vi "test Add Invalid Alias.vi"(8 "error in (no error)":errorcluster, 11 "TestCase in":refnum<class "Routing and Faulting Aliases Unit Tests.lvclass">) -> (0 "error out":errorcluster, 3 "TestCase out":refnum<class "Routing and Faulting Aliases Unit Tests.lvclass">)   [LabVIEW 2019, in "Routing and Faulting Aliases Unit Tests.lvclass"]
uses:
  Routing and Faulting Aliases Unit Tests.lvclass
  Shared/Alias Mapping.ctl
  Shared/Alias Endpoint.ctl
  System Explorer/Alias.ctl
  System Explorer/Endpoint.ctl
  Routing and Faulting Aliases Unit Tests.lvclass/Routing and Faulting Aliases Unit Tests.ctl
  <vilib>/addons/_JKI Toolkits/VI Tester/TestCase.llb/TestCase.lvclass
  System Explorer/Routing and Faulting System Explorer.lvlib
  Scripting/Routing and Faulting Scripting.lvlib
  Shared/Routing and Faulting Shared.lvlib
  C:/Program Files (x86)/National Instruments/LabVIEW 2019/vi.lib/addons/_JKI Toolkits/VI Tester/TestCase.llb/TestCase.lvclass
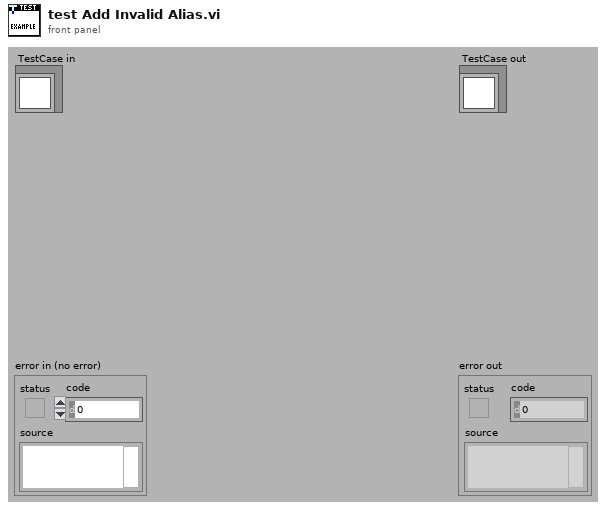
[diagram p1: front panel]
types:
  T1 = typedef "Routing and Faulting Shared.lvlib/Alias Endpoint.ctl" = cluster{"Module Path":string, "Endpoint":string}
  T2 = typedef "Routing and Faulting System Explorer.lvlib/Endpoint.ctl" = string
  T3 = typedef "Routing and Faulting Shared.lvlib/Alias Mapping.ctl" = cluster{"Alias":string, "Endpoint":T1}
  T4 = typedef "Routing and Faulting System Explorer.lvlib/Alias.ctl" = cluster{"Endpoint":T2, "Alias":string, "Remove":bool}
  T5 = typedef "Custom Device API.lvlib/Custom Device Item Ref.ctl" = u64
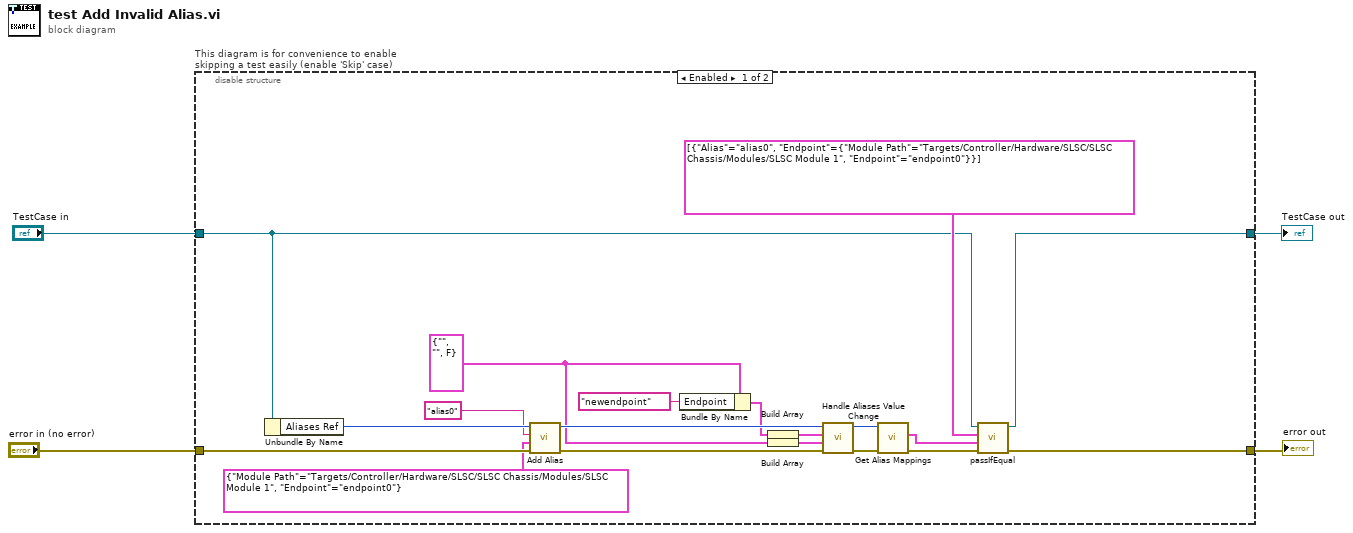
[diagram p0: block diagram]
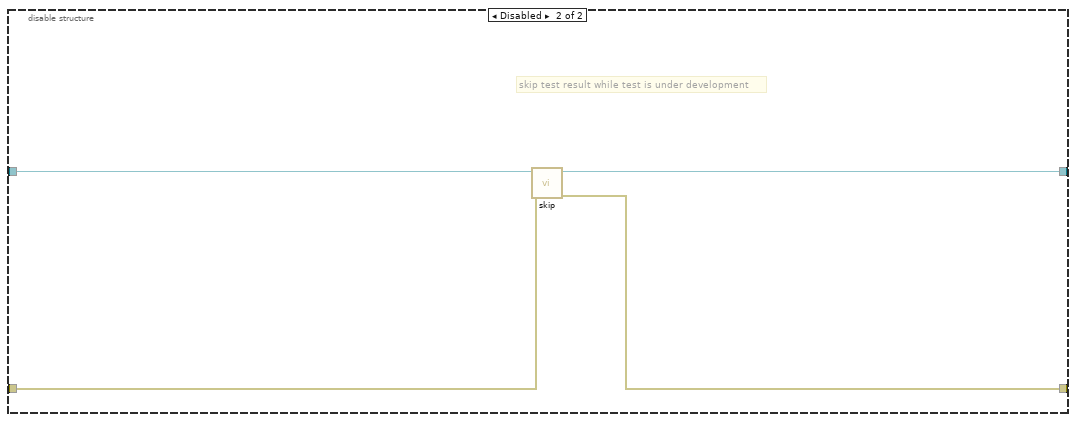
[diagram p2: hidden frame]
diagram:
  n1 = disable-structure "This diagram is for convenience to enable skipping a test easily (enable 'Skip' case)" shown="Enabled" {
    disable-tunnel: "TestCase in" -> [w17 w27]
    disable-tunnel: [w16 w25] -> w1
    disable-tunnel: [w20 w26] -> w3
    disable-tunnel: "error in (no error)" -> [w14 w24]
    frame Enabled {
      w7 = T4 {"Endpoint"="", "Alias"="", "Remove"=FALSE} ("Alias")
      n2 = Unbundle By Name(w17) -> ("Aliases Ref"=w15:T5)
      n3 = call "Add Alias.vi"("error in"=w14, "endpoint"=T1 {"Module Path"="Targets/Controller/Hardware/SLSC/SLSC Chassis/Modules/SLSC Module 1", "Endpoint"="endpoint0"} ("Endpoint"), "alias"="alias0" ("Alias"), "endpoint aliases in"=w15) -> ("error out"=w12:errorcluster, "endpoint aliases out"=w13:T5)  [unwired: 6 in]
      n4 = Bundle By Name(cluster=w7, "Endpoint"=T2 "newendpoint") -> (w8:T4)
      n5 = Build Array(w8) -> (w9:T4[])
      n6 = Build Array(w7) -> (w10:T4[])
      n7 = call "Handle Aliases Value Change.vi"("error in (no error)"=w12, "OldVal"=w10, "NewVal"=w9, "Aliases Ref in"=w13) -> ("error out"=w23:errorcluster, "Aliases Ref out"=w22:T5)  [unwired: 4 in, 2 out]
      n8 = call "Get Alias Mappings.vi"("error in"=w23, "endpoint aliases in"=w22) -> ("error out"=w21:errorcluster, "alias mappings"=w19:T3[])  [unwired: 7 in, 1 out]
      n9 = call-dynamic "passIfEqual.vi"("error in (no error)"=w21, "y"=w19, "x"=T3[] [{"Alias"="alias0", "Endpoint"={"Module Path"="Targets/Controller/Hardware/SLSC/SLSC Chassis/Modules/SLSC Module 1", "Endpoint"="endpoint0"}}] ("Alias Mappings"), "TestCase in"=w17) -> ("error out"=w20:errorcluster, "TestCase out"=w16:refnum<class "Routing and Faulting Aliases Unit Tests.lvclass">)  [unwired: 6 in]
    }
    frame Disabled {
      # "skip test result while test is under development"
      n10 = call <vilib>:"skip.vi"("error in (no error)"=w24, "TestCase in"=w27) -> ("error out"=w26:errorcluster, "TestCase out"=w25:refnum<class "Routing and Faulting Aliases Unit Tests.lvclass">)  [unwired: 8 in]
    }
  }
  "error out" <- w3
  "TestCase out" <- w1
